vi "Unpack Auto-Launch Nested Models.vi"(11 "Launch Nested Models Msg":refnum<class "Auto-Launch Models Msg.lvclass">) -> (0 "Confirm Shutdown? (T)":bool=TRUE, 1 "Auto-stop? (T)":bool=TRUE, 2 "Nested Models":refnum<class "IModel.lvclass">[](array[class]))   [LabVIEW 2020, in "MVA Framework.lvlib" / "IModel.lvlib" / "Auto-Launch Models Msg.lvclass"]
uses:
  Auto-Launch Models Msg.lvclass
  IModel/IModel.lvclass
  Auto-Launch Models Msg.lvclass/Auto-Launch Models Msg.ctl
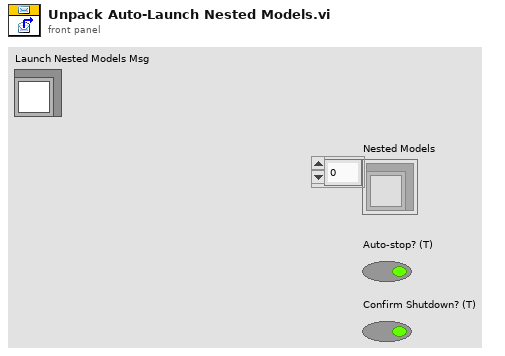
[diagram p1: front panel]
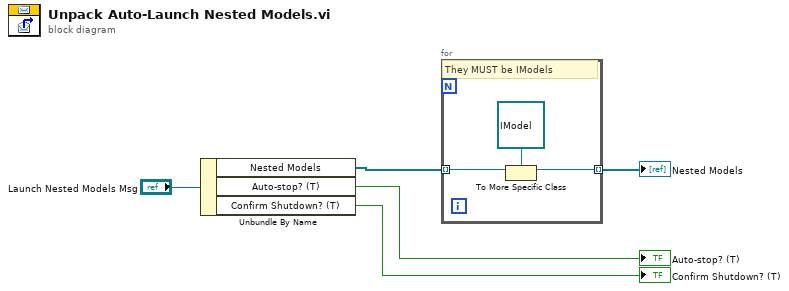
[diagram p0: block diagram]
diagram:
  n1 = Unbundle By Name("Launch Nested Models Msg") -> ("Nested Models"=w4:refnum<class "Actor.lvclass">[], "Auto-stop? (T)"=→"Auto-stop? (T)":bool, "Confirm Shutdown? (T)"=→"Confirm Shutdown? (T)":bool)
  n2 = for {
    tunnel: w4 -> [w8] mode=indexing
    tunnel: [w7] -> w3 mode=indexing
    # "They MUST be IModels"
    n3 = To More Specific Class(target class=refnum<class "IModel.lvclass"> refnum ("IModel.lvlib:IModel.lvclass"), reference=w8) -> (specific class reference=w7:refnum<class "IModel.lvclass">)  [unwired: 1 in, 1 out]
  }
  "Nested Models" <- w3
